vi "Cartesian to polar and Rotate vector.vi"(1 "Angle":dbl, 2 "Cluster":T2) -> (0 "output cluster":T1)   [LabVIEW 2014]
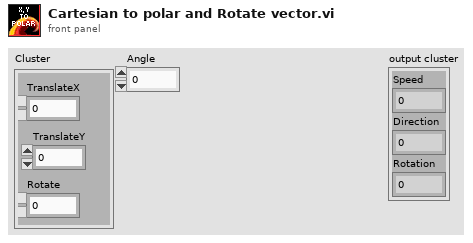
[diagram p1: front panel]
types:
  T1 = cluster{"Speed":dbl, "Direction":dbl, "Rotation":dbl}
  T2 = cluster{"TranslateX":dbl, "TranslateY":dbl, "Rotate":dbl}
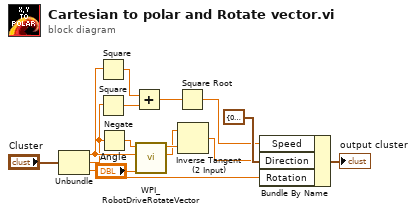
[diagram p0: block diagram]
diagram:
  n1 = Unbundle("Cluster") -> ("TranslateX"=w8:dbl, "TranslateY"=w7:dbl, "Rotate"=w3:dbl)
  n2 = Square(x=w8) -> (x^2=w14:dbl)
  n3 = Square(x=w7) -> (x^2=w15:dbl)
  n4 = Negate(x=w7) -> (-x=w10:dbl)
  n5 = Add(x=w14, y=w15) -> (x+y=w13:dbl)
  n6 = call <vilib>:"WPI_RobotDriveRotateVector.vi"("Angle"="Angle", "X"=w8, "Y"=w10) -> ("X'"=w11:dbl, "Y'"=w12:dbl)  [unwired: 7 out]
  n7 = Square Root(x=w13) -> (sqrt(x)=w5:dbl)
  n8 = Inverse Tangent (2 Input)(1:w12, 2:w11) -> (0:w4:dbl)
  n9 = Bundle By Name(cluster=T1 {"Speed"=0.0, "Direction"=0.0, "Rotation"=0.0} ("Drive Controls"), "Speed"=w5, "Direction"=w4, "Rotation"=w3) -> (→"output cluster":T1)
